vi "Insight_Discovery.vi"(8 "error in (no error)":errorcluster) -> (0 "error out":errorcluster, 3 "Available Lasers":T1(array[cluster]))   [LabVIEW 2014]
panel:
  out "error out (discovery)":errorcluster
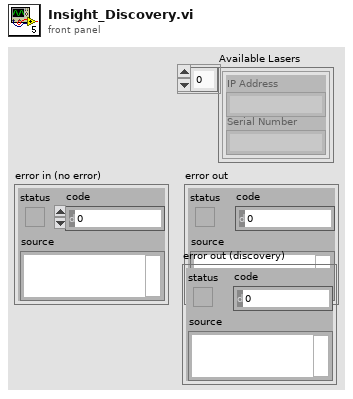
[diagram p1: front panel]
types:
  T1 = cluster{"IP Address":string, "Serial Number":string}[]
  T2 = cluster{"IP Address":string, "Serial Number":string}
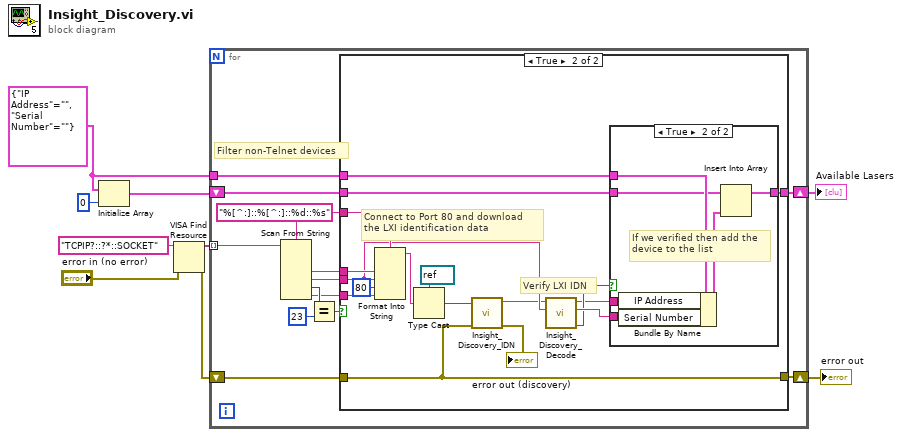
[diagram p0: block diagram]
diagram:
  w5 = T2 {"IP Address"="", "Serial Number"=""}
  n1 = Initialize Array(w5, 0 ("dimension size")) -> (w7:T1)
  n2 = VISA Find Resource(8:"error in (no error)", 11:"TCPIP?::?*::SOCKET" ("expression (\"?*\")")) -> (0:w3:errorcluster, 3:w8:string[])  [unwired: 1 in, 1 out]
  n3 = for {
    tunnel: w8 -> [w19] mode=indexing
    shift-right: [w10] -> w4
    shift-left: w7 -> [w14]
    tunnel: w5 -> [w13]
    shift-right: [w11] -> w2
    shift-left: w3 -> [w12]
    w20 = "%[^:]::%[^:]::%d::%s" ("format string")
    # "Filter non-Telnet devices"
    n4 = Scan From String(format string=w20, input string=w19) -> (output 1=w18:string, output 2=w17:string, output 3=w22:i32, output 4=w16:string)  [unwired: 6 in, 3 out]
    n5 = Equal?(x=w22, y=23) -> (x = y?=w15:bool)
    n6 = case shown="True" w15 {
      tunnel: w20 -> [_ w40]
      tunnel: w18 -> [_ w39]
      tunnel: w17 -> [_ w34]
      tunnel: w16 -> [_ w38]
      tunnel: w14 -> [w23 w29]
      tunnel: w13 -> [_ w30]
      tunnel: w12 -> [w24 w26]
      tunnel: [w24 w26] -> w11
      tunnel: [w23 w28] -> w10
      frame False {
      }
      frame True {
        # "Verify LXI IDN"
        # "Connect to Port 80 and download\nthe LXI identification data"
        n7 = Format Into String(format string=w40, w39, w34, 80 ("input 3"), w38) -> (resulting string=w37:string)  [unwired: 2 in, 1 out]
        n8 = Type Cast(type=refnum<visa-resource-name> refnum ("VISA resource name"), x=w37) -> (*(type *) &x=w35:refnum<visa-resource-name>)
        n9 = call "Insight_Discovery_IDN.vi"("error in (no error)"=w26, "VISA resource name"=w35) -> ("error out"=→"error out (discovery)":errorcluster, "IDN"=w33:string)  [unwired: 8 in]
        n10 = call "Insight_Discovery_Decode.vi"("IP Address (in)"=w34, "IDN"=w33) -> ("Succeeded"=w31:bool, "Serial Number"=w32:string, "IP Address (out)"=w27:string)  [unwired: 7 in]
        n11 = case shown="True" w31 {
          tunnel: w27 -> [_ w48]
          tunnel: w32 -> [_ w47]
          tunnel: w30 -> [_ w46]
          tunnel: w29 -> [w42 w45]
          tunnel: [w42 w44] -> w28
          frame False {
          }
          frame True {
            # "If we verified then add the\ndevice to the list"
            n12 = Bundle By Name(cluster=w46, "IP Address"=w48, "Serial Number"=w47) -> (w43:T2)
            n13 = Insert Into Array(array=w45, new element=w43) -> (w44:T1)  [unwired: 1 in]
          }
        }
      }
    }
  }
  "Available Lasers" <- w4
  "error out" <- w2
